vi "DangerZone(ElevatorWrist)ARCHIVE.vi"(3 "Wrist":T2(ring), 5 "Level":T1(ring)) -> (0 "Wrist":T2(ring), 1 "Park Horse":bool=TRUE, 2 "Level":T1(ring))   [LabVIEW 2018]
uses:
  <vilib>/Rock Robotics/WPI/ThirdParty/Phoenix-LabVIEW/Motor Controller/Get/CTRE_Phoenix_MotorController_GetSelectedSensorData.vi
panel:
  in  "Horse Upper Danger":i32
  in  "Horse Lower Danger":i32
  in  "Intake Lower Danger":i32
  in  "Intake Upper Danger":i32
  in  "Elevator Lower Danger":i32
  in  "Elevator Upper Danger":i32
  in  "Intake Upper Danger GO TO Cargoship Back":i32
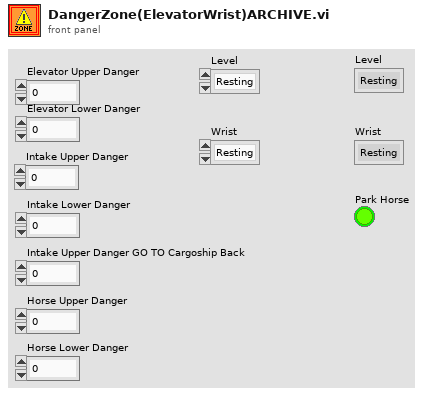
[diagram p1: front panel]
types:
  T1 = enum16{"Resting", "CargoShip Front", "CargoShip Back", "Cargo Mid", "Hatch Mid", "All High"}
  T2 = enum16{"Resting", "Hatch Ground Intake", "Hatch Place Low/Mid/CargoShip", "Hatch Place High", "Cargo Ground Intake", "Cargo Place Low/Mid", "Cargo Place High", "CargoShip Place Front", "CargoShip Place Back"}
  T3 = typedef "WPI_MotorControlDeviceRef.ctl" = cluster{"DeviceStatus":errorcluster, "Type":T4, "PWM":cluster{"PWM Channel":T5, "DeadBand":T6}, "CAN":cluster{"Device Number":u8, "SetOutput VI Ref":variant, "GetOutput VI Ref":variant, "Enable VI Ref":variant, "Disable VI Ref":variant, "Data":variant}, "Invert":bool, "DIO PWM":cluster{"PWM \"Enable\" Channel":T5, "DIOChannel":T7, "PWM Rate":dbl}}
  T4 = typedef "WPI_MotorControlType.ctl" = enum16{"PWM", "CAN", "DIO PWM"}
  T5 = typedef "FPGA_DIOPWMChannel.ctl" = enum8{"PWM 0", "PWM 1", "PWM 2", "PWM 3", "PWM 4", "PWM 5", "PWM 6", "PWM 7", "PWM 8", "PWM 9", "PWM MXP 0", "PWM MXP 1", "PWM MXP 2", "PWM MXP 3", "PWM MXP 4", "PWM MXP 5", "PWM MXP 6", "PWM MXP 7", "PWM MXP 8", "PWM MXP 9", "Invalid"}
  T6 = typedef "WPI_PWMDeadband.ctl" = cluster{"Name":string, "maxPositivePwm":i32, "minPositivePwm":i32, "centerPwm":i32, "maxNegativePwm":i32, "minNegativePwm":i32, "angularRange":u16}
  T7 = typedef "FPGA_DIOChannel.ctl" = enum8{"DIO 0", "DIO 1", "DIO 2", "DIO 3", "DIO 4", "DIO 5", "DIO 6", "DIO 7", "DIO 8", "DIO 9", "DIO MXP 0", "DIO MXP 1", "DIO MXP 2", "DIO MXP 3", "DIO MXP 4", "DIO MXP 5", "DIO MXP 6", "DIO MXP 7", "DIO MXP 8", "DIO MXP 9", "DIO MXP 10", "DIO MXP 11", "DIO MXP 12", "DIO MXP 13", "DIO MXP 14", "DIO MXP 15", "SPI Port CS1", "SPI Port CS2", "SPI Port CS3", "SPI Port MISO", "SPI Port MOSI", "Invalid"}
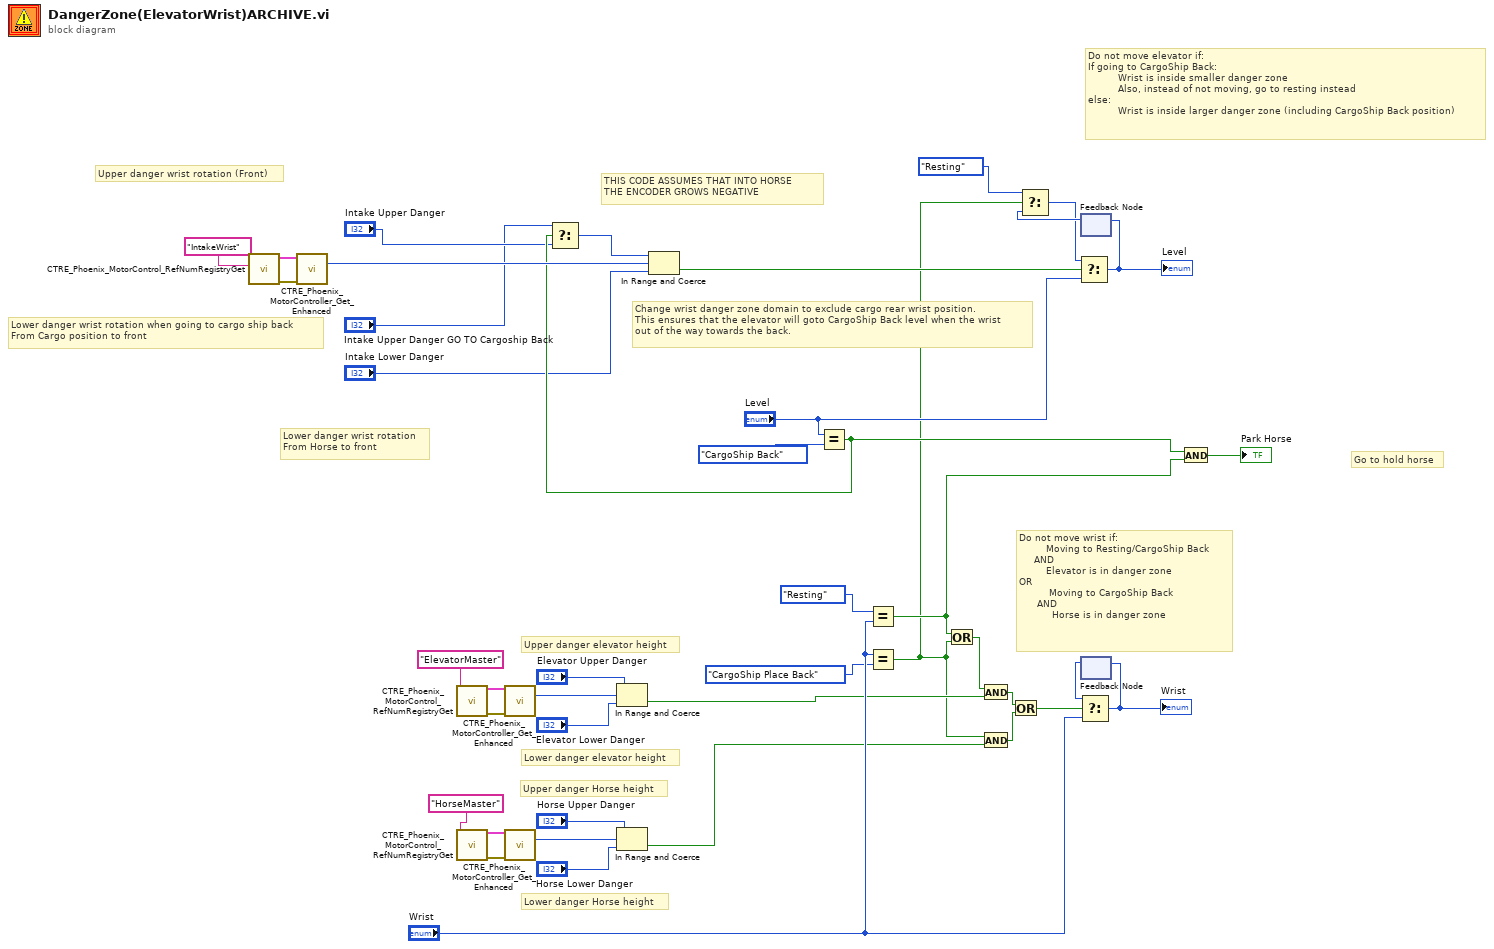
[diagram p0: block diagram]
diagram:
  # "Go to hold horse"
  # "Do not move elevator if:\nIf going to CargoShip Back:\n          Wrist is inside smaller danger zone\n          Also, instead of not moving, go to resting instead\nelse:\n          Wrist is inside larger danger zone (including CargoShip Back position)"
  # "Do not move wrist if:\n         Moving to Resting/CargoShip Back\n     AND\n         Elevator is in danger zone\nOR\n          Moving to CargoShip Back\n      AND\n           Horse is in danger zone"
  # "Lower danger Horse height"
  # "Upper danger Horse height"
  # "Change wrist danger zone domain to exclude cargo rear wrist position.\nThis ensures that the elevator will goto CargoShip Back level when the wrist\nout of the way towards the back."
  # "THIS CODE ASSUMES THAT INTO HORSE\nTHE ENCODER GROWS NEGATIVE"
  # "Lower danger wrist rotation when going to cargo ship back\nFrom Cargo position to front"
  # "Lower danger elevator height"
  # "Upper danger wrist rotation (Front)"
  # "Lower danger wrist rotation\nFrom Horse to front"
  # "Upper danger elevator height"
  n1 = call <vilib>:"CTRE_Phoenix_MotorControl_RefNumRegistryGet.vi"("refnum name"="IntakeWrist") -> ("error out"=w41:errorcluster, "PhoenixMotorControlDevRef"=w40:T3)  [unwired: 9 in]
  n2 = call-poly <vilib>:"CTRE_Phoenix_MotorController_Get_Enhanced.vi"("PhoenixMotorControlDevRef"=w40, "error in"=w41) -> ("Position (Raw Sensor Units)"=w39:i32)  [unwired: 10 in, 3 out]
  n3 = call <vilib>:"CTRE_Phoenix_MotorControl_RefNumRegistryGet.vi"("refnum name"="ElevatorMaster") -> ("error out"=w37:errorcluster, "PhoenixMotorControlDevRef"=w36:T3)  [unwired: 9 in]
  n4 = call <vilib>:"CTRE_Phoenix_MotorControl_RefNumRegistryGet.vi"("refnum name"="HorseMaster") -> ("error out"=w20:errorcluster, "PhoenixMotorControlDevRef"=w21:T3)  [unwired: 9 in]
  n5 = call-poly <vilib>:"CTRE_Phoenix_MotorController_Get_Enhanced.vi"("PhoenixMotorControlDevRef"=w36, "error in"=w37) -> ("Position (Raw Sensor Units)"=w35:i32)  [unwired: 10 in, 3 out]
  n6 = call-poly <vilib>:"CTRE_Phoenix_MotorController_Get_Enhanced.vi"("PhoenixMotorControlDevRef"=w21, "error in"=w20) -> ("Position (Raw Sensor Units)"=w22:i32)  [unwired: 10 in, 3 out]
  n7 = In Range and Coerce(upper limit="Elevator Upper Danger", x=w35, lower limit="Elevator Lower Danger") -> (In Range?=w9:bool)  [unwired: 1 out]
  n8 = In Range and Coerce(upper limit="Horse Upper Danger", x=w22, lower limit="Horse Lower Danger") -> (In Range?=w11:bool)  [unwired: 1 out]
  n9 = Equal?(x="Level", y=T1."CargoShip Back" ("f")) -> (x = y?=w15:bool)
  n10 = Select(t="Intake Upper Danger GO TO Cargoship Back", s=w15, f="Intake Upper Danger") -> (s? t:f=w4:i32)
  n11 = In Range and Coerce(upper limit=w4, x=w39, lower limit="Intake Lower Danger") -> (In Range?=w25:bool)  [unwired: 1 out]
  n12 = Equal?(x=T2."Resting" ("Wrist 2"), y="Wrist") -> (x = y?=w14:bool)
  n13 = Equal?(x="Wrist", y=T2."CargoShip Place Back" ("Wrist 2")) -> (x = y?=w5:bool)
  n14 = Or(x=w14, y=w5) -> (x .or. y?=w10:bool)
  n15 = And(x=w10, y=w9) -> (x .and. y?=w8:bool)
  n16 = And(x=w5, y=w11) -> (x .and. y?=w7:bool)
  n17 = Or(x=w8, y=w7) -> (x .or. y?=w6:bool)
  n18 = feedback #1() -> (w27:T1)  [unwired: 1 in]
  n19 = Select(t=T1."Resting" ("f"), s=w5, f=w27) -> (s? t:f=w26:T1)
  n20 = Select(t=w26, s=w25, f="Level") -> (s? t:f=w32:T1)
  "Level" <- w32
  n21 = feedback-in #1(w32) -> ()
  n22 = feedback #2() -> (w30:T2)  [unwired: 1 in]
  n23 = Select(t=w30, s=w6, f="Wrist") -> (s? t:f=w31:T2)
  "Wrist" <- w31
  n24 = feedback-in #2(w31) -> ()
  n25 = And(x=w15, y=w14) -> (x .and. y?=→"Park Horse":bool)
